vi "_Read.vi"(8 "error in (no error)":errorcluster, 10 "Count":i32, 11 "FileStream in":refnum<class "FileStream.lvclass">) -> (0 "error out":errorcluster, 2 "Data":string, 3 "FileStream out":refnum<class "FileStream.lvclass">, 5 "Message ID":string)   [LabVIEW 2020, in "Stream.lvlib" / "FileStream.lvclass"]
uses:
  FileStream.lvclass
  C:/dev/IlluminatedG/lv-stream/stream/Stream/Stream.lvclass
  FileStream.lvclass/FileStream.ctl
  Message.ctl
  Stream/Stream.lvclass
  Stream.lvlib
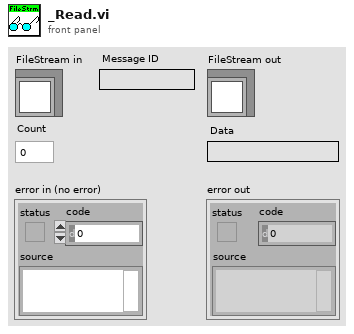
[diagram p1: front panel]
types:
  T1 = typedef "Stream.lvlib/Mode.ctl" = enum16{"Raw", "Buffered", "LineTerm", "Message"}
  T2 = typedef "Stream.lvlib/Message.ctl" = cluster{"id":string, "data":string}
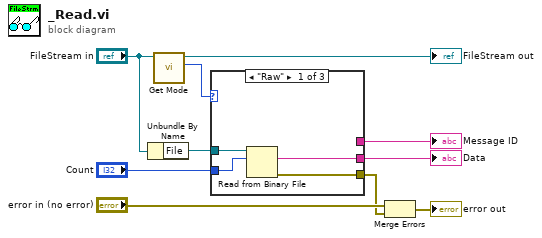
[diagram p0: block diagram]
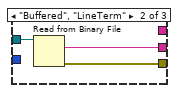
[diagram p2: hidden frame]
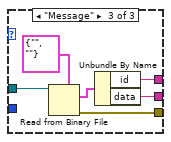
[diagram p3: hidden frame]
diagram:
  n1 = Unbundle By Name("FileStream in") -> ("File"=w9:refnum<file>)
  n2 = call "Get Mode.vi"("Stream in"="FileStream in") -> ("Mode"=w3:T1, "Stream out"=→"FileStream out":refnum<class "FileStream.lvclass">)  [unwired: 8 in, 1 out]
  n3 = case shown="\"Raw\"" w3 {
    tunnel: w9 -> [w14 w15 w23]
    tunnel: "Count" -> [w13 _ _]
    tunnel: [w12 w17 w19] -> w7
    tunnel: [w11 w16 w22] -> w5
    tunnel: [_ _ w18] -> w2
    frame "Raw" {
      n4 = Read from Binary File(10:w13, 11:w14) -> (0:w11:errorcluster, 2:w12:string)  [unwired: 4 in, 2 out]
    }
    frame "Buffered", "LineTerm" {
      n5 = Read from Binary File(11:w15) -> (0:w16:errorcluster, 2:w17:string)  [unwired: 5 in, 2 out]
    }
    frame "Message" {
      n6 = Read from Binary File(5:T2 {"id"="", "data"=""} ("Message"), 11:w23) -> (0:w22:errorcluster, 2:w20:T2)  [unwired: 4 in, 2 out]
      n7 = Unbundle By Name(w20) -> ("id"=w18:string, "data"=w19:string)
    }
  }
  "Data" <- w7
  "Message ID" <- w2
  n8 = Merge Errors("error in (no error)", w5) -> (→"error out":errorcluster)
